vi "MedianFilter_Reset.vi"(11 "In MEDIAN_FILTER":T1 {"ValueBuffer" format="%13.5g"}) -> (3 "Out MEDIAN_FILTER":T1 {"ValueBuffer" format="%13.5g"})   [LabVIEW 2019, in "Trajectory_Library.lvlib"]
doc: "Resets the filter, clearing the window of all elements. All stored values are set to zero.\n\nInputs:\n - In Median Filter -- Median filter data structure\n\nOutputs:\n - Out Median Filter -- Updated median filter data structure"
uses:
  Trajectory_Library.lvlib
  TypeDef/MEDIAN_FILTER.ctl
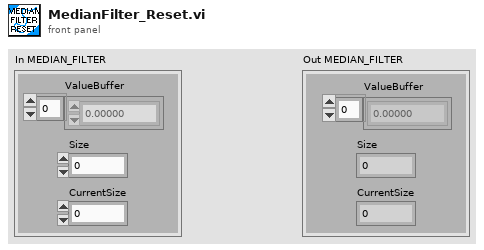
[diagram p1: front panel]
types:
  T1 = typedef "Trajectory_Library.lvlib/MEDIAN_FILTER.ctl" = cluster{"ValueBuffer":dbl[], "Size":i32, "CurrentSize":i32}
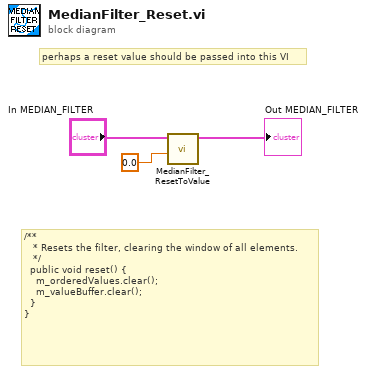
[diagram p0: block diagram]
diagram:
  # "perhaps a reset value should be passed into this VI"
  # "/**\n   * Resets the filter, clearing the window of all elements.\n   */\n  public void reset() {\n    m_orderedValues.clear();\n    m_valueBuffer.clear();\n  }\n}"
  n1 = call "MedianFilter_ResetToValue.vi"("Value"=0.0, "In MEDIAN_FILTER"="In MEDIAN_FILTER") -> ("Out MEDIAN_FILTER"=→"Out MEDIAN_FILTER":T1)  [unwired: 9 in]
